vi "Config_File_Path.vi"() -> (2 "Config File Path":path)   [LabVIEW 2024]
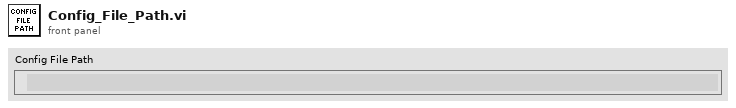
[diagram p1: front panel]
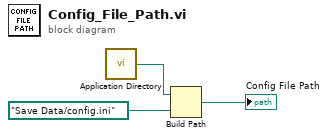
[diagram p0: block diagram]
diagram:
  n1 = call <vilib>:"Application Directory.vi"() -> ("Application Directory"=w2:path)
  n2 = Build Path(base path=w2, name or relative path=path "Save Data/config.ini") -> (appended path=→"Config File Path":path)
